vi "创建数据表.vi"(8 "error in (no error)":errorcluster) -> (0 "error out":errorcluster)   [LabVIEW 2016, in "数据查询.lvlib"]
uses:
  <vilib>/addons/database/Auxilliary.llb/DB Tools Column Info.ctl
  <vilib>/addons/database/Auxilliary.llb/DB Tools DataTypes.ctl
  <vilib>/addons/database/Connection.llb/DB Tools Open Connec (String).vi
  <userlib>/_LVST/sqlite_api/Core/Tables/SQLite_Drop Table.vi
  <userlib>/_LVST/sqlite_api/Core/Tables/SQLite_Create Table.vi
  <vilib>/addons/database/NI_Database_API.lvlib
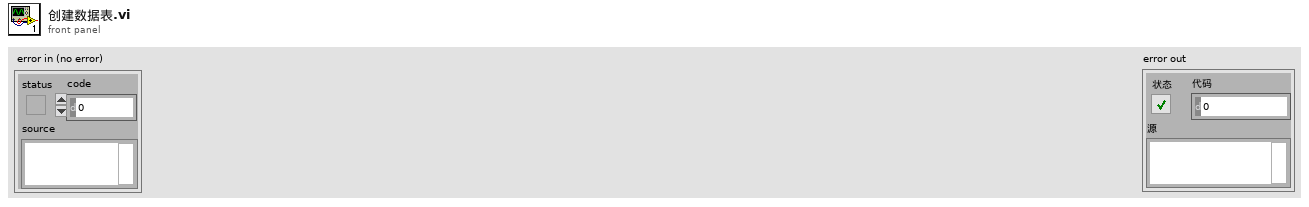
[diagram p1: front panel]
types:
  T1 = typedef "数据库类型.ctl" = enum16{"Access", "SQLite"}
  T2 = typedef "NI_Database_API.lvlib/DB Tools Column Info.ctl" = cluster{"column name":string, "data type":T3, "size":i32, "allow null?":bool}
  T3 = typedef "NI_Database_API.lvlib/DB Tools DataTypes.ctl" = enum16{"String", "Long (I32)", "Single (SGL)", "Double (DBL)", "Date/Time", "Binary"}
  T4 = typedef "NI_Database_API.lvlib/Conn ObjectReference.ctl" = refnum<k1>
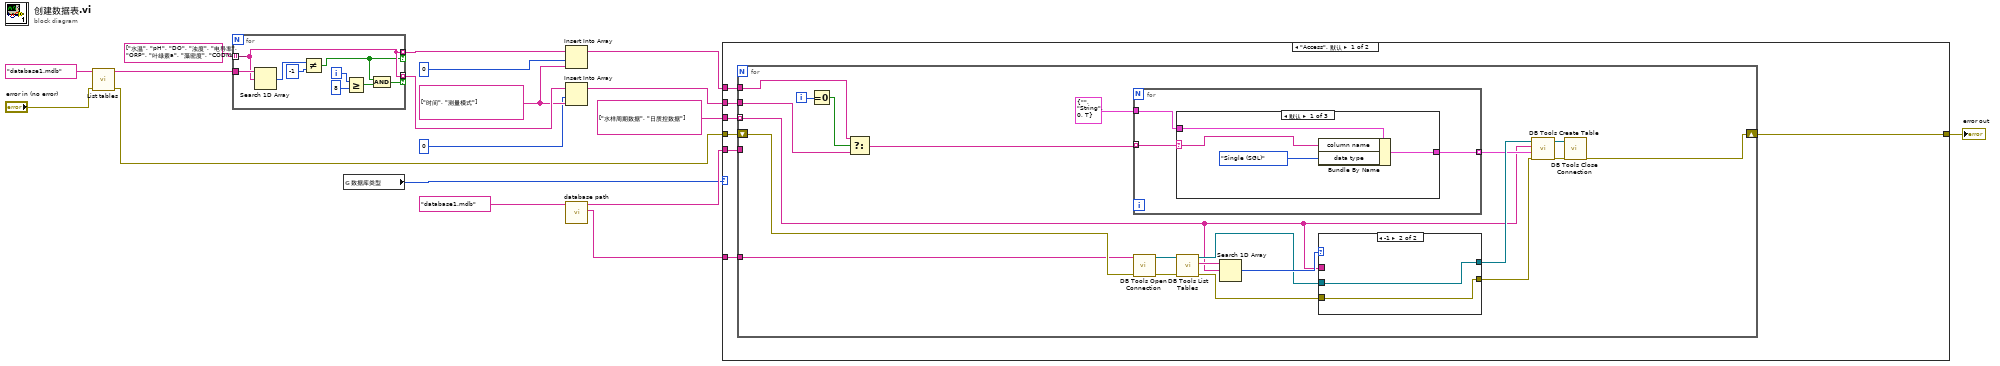
[diagram p0: block diagram]
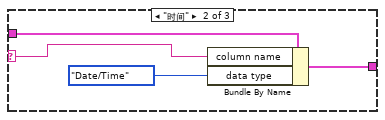
[diagram p2: hidden frame]
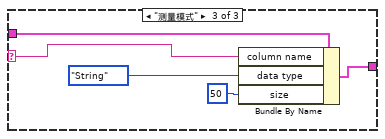
[diagram p3: hidden frame]
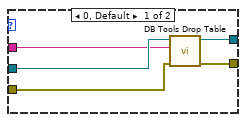
[diagram p4: hidden frame]
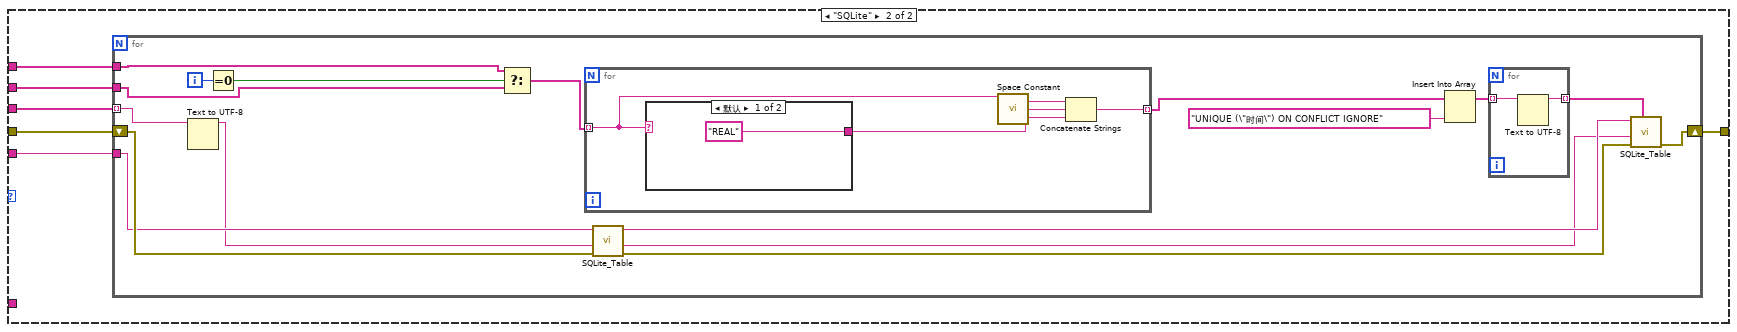
[diagram p5: hidden frame]
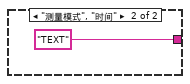
[diagram p6: hidden frame]
diagram:
  w13 = string[] ["时间", "测量模式"]
  n1 = call "List tables.vi"("error in (no error)"="error in (no error)", "database"="database1.mdb") -> ("error out"=w10:errorcluster, "tables"=w18:string[])  [unwired: 8 in]
  n2 = for {
    tunnel: string[] ["水温", "pH", "DO", "浊度", "电导率", "ORP", "叶绿素a", "藻密度", "CODMn", "CODcr", "COD", "磷酸盐", "氨氮", "总磷", "总氮", "亚硝氮", "硫化物", "硝氮", "硅酸盐"] -> [w24] mode=indexing
    tunnel: w18 -> [w27]
    tunnel: [w24] -> w17 mode=indexing if=w19
    tunnel: [w24] -> w14 mode=indexing if=w20
    i -> [w23]
    n3 = Search 1D Array(1D array=w27, element=w24) -> (index of element=w26:i32)  [unwired: 1 in]
    n4 = Not Equal?(x=w26, y=-1 ("x")) -> (x != y?=w19:bool)
    n5 = Greater Or Equal?(x=w23, y=8) -> (x >= y?=w21:bool)
    n6 = And(x=w19, y=w21) -> (x .and. y?=w20:bool)
  }
  n7 = global read "外部调用接口全局变量.vi" "数据库类型"() -> (w1:T1)
  n8 = Insert Into Array(array=w17, index=0 ("索引"), new element=w13) -> (w9:string[])
  n9 = Insert Into Array(array=w14, index=0 ("索引"), new element=w13) -> (w7:string[])
  n10 = call "database path.vi"("database"="database1.mdb") -> ("Connection information"=w2:string, "Path out"=w3:string)  [unwired: 9 in]
  n11 = case shown="\"Access\", 默认" w1 {
    tunnel: w9 -> [w34 w83]
    tunnel: w10 -> [w33 w80]
    tunnel: [w32 w81] -> w5
    tunnel: string[] ["水样周期数据", "日质控数据"] -> [w31 w84]
    tunnel: w7 -> [w30 w82]
    tunnel: w3 -> [w29 w79]
    tunnel: w2 -> [w28 _]
    frame "Access", Default {
      n12 = for {
        tunnel: w34 -> [w38]
        shift-right: [w42] -> w32
        shift-left: w33 -> [w43]
        tunnel: w31 -> [w41] mode=indexing
        tunnel: w30 -> [w37]
        tunnel: w29 -> [_]
        tunnel: w28 -> [w35]
        i -> [w40]
        n13 = Equal To 0?(x=w40) -> (x = 0?=w39:bool)
        n14 = Select(t=w38, s=w39, f=w37) -> (s? t:f=w36:string[])
        n15 = for {
          tunnel: w36 -> [w58] mode=indexing
          tunnel: T2 {"column name"="", "data type"=enum."String", "size"=0, "allow null?"=TRUE} ("column information") -> [w57]
          tunnel: [w56] -> w44 mode=indexing
          n16 = case shown="默认" w58 {
            selector: w58 -> [w61 w65 w70]
            tunnel: w57 -> [w62 w66 w71]
            tunnel: [w60 w64 w69] -> w56
            frame Default {
              n17 = Bundle By Name(cluster=w62, "column name"=w61, "data type"=DB_Tools_DataTypes."Single (SGL)") -> (w60:T2)
            }
            frame "时间" {
              n18 = Bundle By Name(cluster=w66, "column name"=w65, "data type"=DB_Tools_DataTypes."Date/Time") -> (w64:T2)
            }
            frame "测量模式" {
              n19 = Bundle By Name(cluster=w71, "column name"=w70, "data type"=DB_Tools_DataTypes."String", "size"=50) -> (w69:T2)
            }
          }
        }
        n20 = call-poly <vilib>:"DB Tools Open Connection.vi"("error in (no error)"=w43, "connection information"=w35) -> ("error out"=w55:errorcluster, "connection reference"=w54:T4)  [unwired: 6 in]
        n21 = call <vilib>:"DB Tools List Tables.vi"("error in (no error)"=w55, "connection reference"=w54) -> ("error out"=w49:errorcluster, "tables"=w53:string[], "connection reference out"=w51:T4)  [unwired: 3 in]
        n22 = Search 1D Array(1D array=w53, element=w41) -> (index of element=w52:i32)  [unwired: 1 in]
        n23 = case shown="-1" w52 {
          tunnel: w51 -> [w76 w78]
          tunnel: [w75 w78] -> w50
          tunnel: w49 -> [w74 w77]
          tunnel: [w73 w77] -> w48
          tunnel: w41 -> [w72 _]
          frame 0, Default {
            n24 = call <vilib>:"DB Tools Drop Table.vi"("error in (no error)"=w74, "table"=w72, "connection reference"=w76) -> ("error out"=w73:errorcluster, "connection reference out"=w75:T4)  [unwired: 5 in]
          }
          frame -1 {
          }
        }
        n25 = call <vilib>:"DB Tools Create Table.vi"("error in (no error)"=w48, "column information"=w44, "table"=w41, "connection reference"=w50) -> ("error out"=w46:errorcluster, "connection reference out"=w47:T4)  [unwired: 4 in]
        n26 = call <vilib>:"DB Tools Close Connection.vi"("error in (no error)"=w46, "connection reference"=w47) -> ("error out"=w42:errorcluster)  [unwired: 5 in]
      }
    }
    frame "SQLite" {
      n27 = for {
        tunnel: w79 -> [w89]
        tunnel: w84 -> [w88] mode=indexing
        tunnel: w83 -> [w96]
        tunnel: w82 -> [w95]
        shift-right: [w93] -> w81
        shift-left: w80 -> [w92]
        i -> [w98]
        n28 = Text to UTF-8(11:w88) -> (3:w87:string)  [unwired: 2 in, 1 out]
        n29 = Equal To 0?(x=w98) -> (x = 0?=w97:bool)
        n30 = Select(t=w96, s=w97, f=w95) -> (s? t:f=w94:string[])
        n31 = for {
          tunnel: w94 -> [w107] mode=indexing
          tunnel: [w104] -> w90 mode=indexing
          n32 = case shown="默认" w107 {
            tunnel: ["REAL" "TEXT"] -> w105
            frame Default {
            }
            frame "测量模式", "时间" {
            }
          }
          n33 = call <vilib>:"Space Constant.vi"() -> ("String"=w106:string)
          n34 = Concatenate Strings(w107, w106, w105) -> (w104:string)
        }
        n35 = call-poly <userlib>:"SQLite_Table.vi"("DB Path"=w89, "Table Name"=w87, "error in (no error)"=w92) -> ("DB Path Out"=w101:string, "Table Name Out"=w99:string, "error out"=w100:errorcluster)  [unwired: 5 in]
        n36 = Insert Into Array(array=w90, new element="UNIQUE (\"时间\") ON CONFLICT IGNORE" ("新元素/子数组")) -> (w86:string[])  [unwired: 1 in]
        n37 = for {
          tunnel: w86 -> [w103] mode=indexing
          tunnel: [w102] -> w85 mode=indexing
          n38 = Text to UTF-8(11:w103) -> (3:w102:string)  [unwired: 2 in, 1 out]
        }
        n39 = call-poly <userlib>:"SQLite_Table.vi"("DB Path"=w101, "Table Name"=w99, "error in (no error)"=w100, "Columns"=w85) -> ("error out"=w93:errorcluster)  [unwired: 4 in, 2 out]
      }
    }
  }
  "error out" <- w5
